vi "play keys.vi"(8 "error in (no error)":errorcluster, 11 "Refnum in":T1) -> (0 "error out":errorcluster)   [LabVIEW 2014]
uses:
  Controls/FPGA Reference.ctl
  Controls/Application Data.vi
  <vilib>/Utility/error.llb/Error Cluster From Error Code.vi
  <vilib>/rvi/errors/niLvFpgaAdjustHostInterfaceError.vi
  <vilib>/rvi/interface/nirviMethod/nirviMethod.xnode
  <vilib>/FPGAPlugInAG/Dynamic/niLvFpga_WriteFifo_Dynamic.vi
  <vilib>/rvi/errors/niLvFpgaMergeErrorWithErrorCode.vi
  <vilib>/FPGAPlugInAG/Dynamic/niLvFpga_ReadFifo_Dynamic.vi
panel:
  out "size(s)":i32
  out "Data":dbl[](graph)
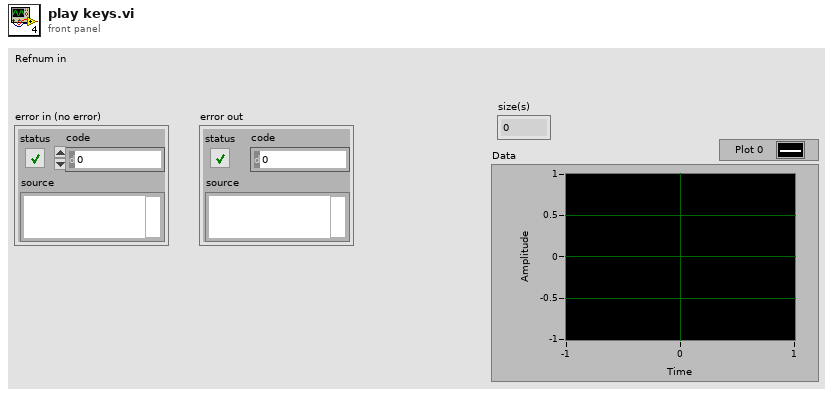
[diagram p1: front panel]
types:
  T1 = typedef "FPGA Reference.ctl" = refnum<k20>
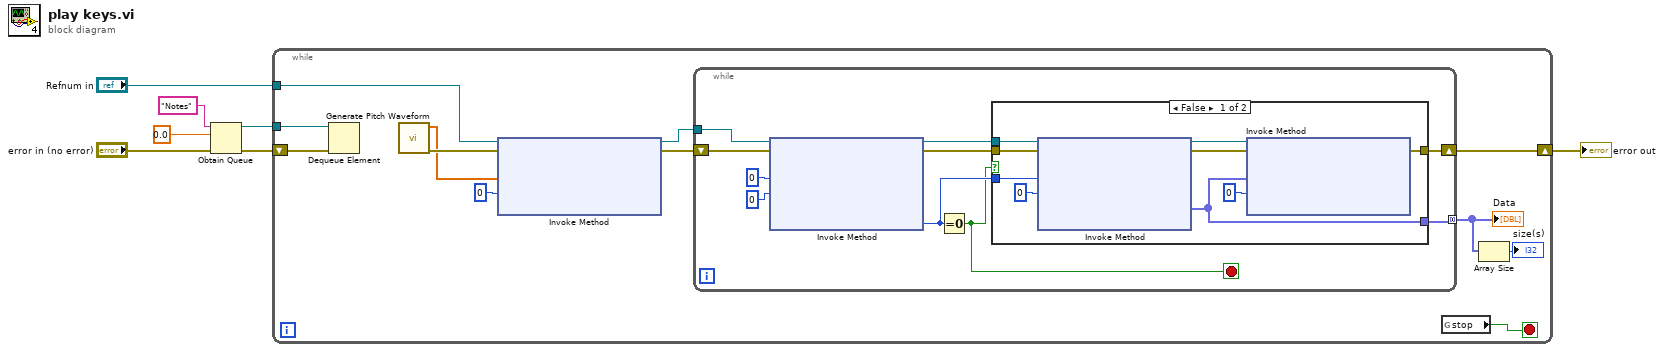
[diagram p0: block diagram]
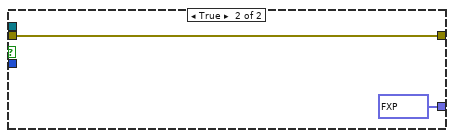
[diagram p2: hidden frame]
diagram:
  n1 = Obtain Queue(name (unnamed)="Notes", element data type=0.0, error in (no error)="error in (no error)") -> (queue out=w2:refnum<queue>, error out=w3:errorcluster)  [unwired: 2 in, 1 out]
  n2 = while {
    tunnel: w2 -> [w15]
    tunnel: "Refnum in" -> [w12]
    shift-right: [w19] -> w7
    shift-left: w3 -> [w16]
    stop <- w11 stop-if-true
    n3 = Dequeue Element(queue=w15, error in (no error)=w16) -> ()  [unwired: 1 in, 4 out]
    n4 = call "Generate Pitch Waveform.vi"() -> ("Error Out"=w17:errorcluster, "Y"=w8:dbl[])  [unwired: 10 in]
    n5 = xnode "Invoke Method"("FPGA VI Reference In"=w12, "error in"=w17, "Data"=w8, "Timeout (ms)"=0) -> ("FPGA VI Reference Out"=w14:T1, "error out"=w18:errorcluster)  [unwired: 1 out]
    n6 = while {
      tunnel: w14 -> [w22]
      shift-right: [w29] -> w19
      shift-left: w18 -> [w28]
      tunnel: [w20] -> w10 mode=concatenating
      stop <- w21 stop-if-true
      n7 = xnode "Invoke Method"("FPGA VI Reference In"=w22, "error in"=w28, "Number of Elements"=u32 0, "Timeout (ms)"=0) -> ("FPGA VI Reference Out"=w23:T1, "error out"=w24:errorcluster, "Elements Remaining"=w25:u32)  [unwired: 1 out]
      n8 = Equal To 0?(x=w25) -> (x = 0?=w21:bool)
      n9 = case shown="False" w21 {
        tunnel: [w38 w40] -> w29
        tunnel: w25 -> [w37 _]
        tunnel: w24 -> [w36 w40]
        tunnel: w23 -> [w35 _]
        tunnel: [w30 fxp<+/-,10,2>[] [0.0] ("Data")] -> w20
        frame False {
          n10 = xnode "Invoke Method"("FPGA VI Reference In"=w35, "error in"=w36, "Number of Elements"=w37, "Timeout (ms)"=0) -> ("FPGA VI Reference Out"=w31:T1, "error out"=w32:errorcluster, "Data"=w30:fxp<+/-,10,2>[])  [unwired: 1 out]
          n11 = xnode "Invoke Method"("FPGA VI Reference In"=w31, "error in"=w32, "Data"=w30, "Timeout (ms)"=0) -> ("error out"=w38:errorcluster)  [unwired: 2 out]
        }
        frame True {
        }
      }
    }
    "Data" <- w10
    n12 = global read "Application Data.vi" "stop"() -> (w11:bool)
    n13 = Array Size(array=w10) -> (size(s)=→"size(s)":i32)
  }
  "error out" <- w7
